vi "STAV wait.vi"(9 "delay (20)":u32=20, 11 "error in (no error)":errorcluster) -> (3 "error out":errorcluster)   [LabVIEW 2021, in "STAV lib.lvlib"]
uses:
  STAV lib.lvlib
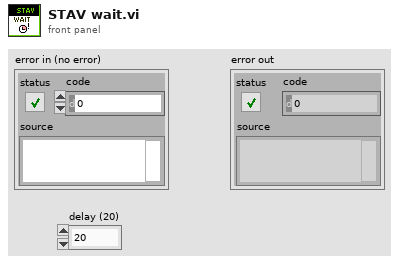
[diagram p1: front panel]
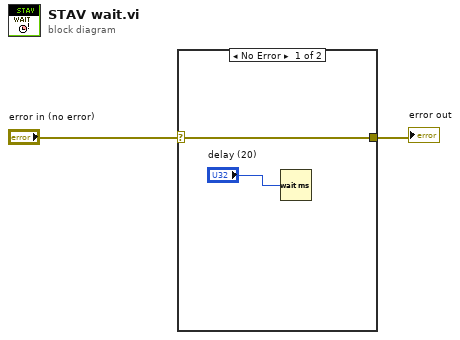
[diagram p0: block diagram]
diagram:
  n1 = case shown="No Error" "error in (no error)" {
    selector: "error in (no error)" -> [w4 w5]
    tunnel: [w4 w5] -> w1
    frame No Error {
      n2 = Wait (ms)(milliseconds to wait="delay (20)") -> ()  [unwired: 1 out]
    }
    frame Error {
    }
  }
  "error out" <- w1
